vi "test_extended_audio.vi"() -> ()   [LabVIEW 2023]
panel:
  out "Waveform Chart":sgl[](graph)
  in  "stop":bool
  in  "host":string="192.168.1.7"
  in  "path in":path=path "C:/Users/jcds/Documents/GitHub/hl2ss/extensions/client_labview/hl2ss_labview/hl2ss_ulm.dll"
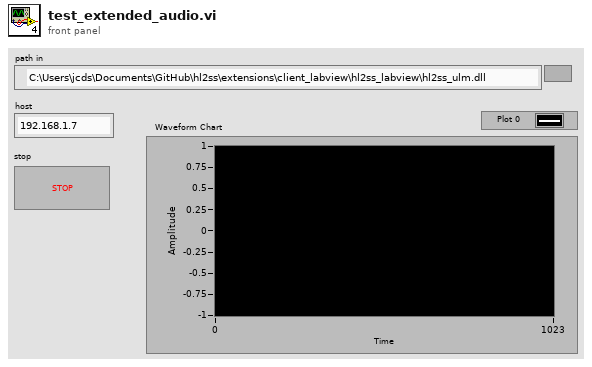
[diagram p1: front panel]
types:
  T1 = cluster{"chunk":u64, "mixer_mode":u32, "loopback_gain":sgl, "microphone_gain":sgl, "profile":u8, "level":u8, "_reserved_0":u8, "_reserved_1":u8}
  T2 = cluster{"frame_stamp":i64, "timestamp":u64, "payload_size":u32, "status":i32, "payload":u64, "pose":u64}
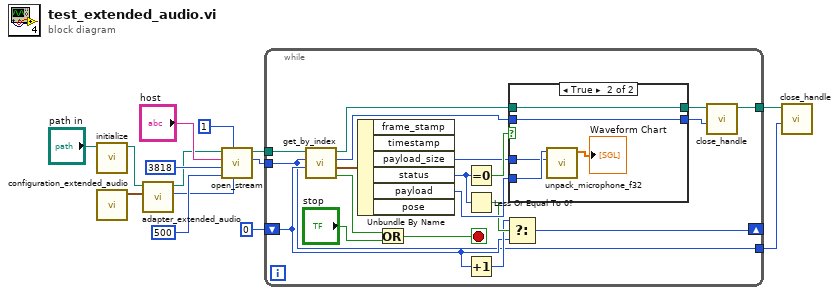
[diagram p0: block diagram]
diagram:
  n1 = call "initialize.vi"("path in"="path in") -> ("path out"=w4:path)  [unwired: 9 in, 1 out]
  n2 = call "configuration_extended_audio.vi"() -> ("configuration_extended_audio"=w5:T1)  [unwired: 11 in]
  n3 = call "adapter_extended_audio.vi"("configuration_extended_audio"=w5, "path in"=w4) -> ("configuration"=w2:u64, "path out"=w3:path)  [unwired: 8 in]
  n4 = call "open_stream.vi"("configuration"=w2, "decoded"=u8 1, "buffer_size"=u64 500, "port"=u16 3818, "host"="host", "path in"=w3) -> ("handle"=w13:u64, "path out"=w12:path)  [unwired: 3 in, 1 out]
  n5 = while {
    shift-right: [w26] -> _
    shift-left: i64 0 ("status") -> [w27]
    tunnel: w13 -> [w19]
    tunnel: w12 -> [w25]
    tunnel: [w20] -> w7
    tunnel: [w19] -> w6
    stop <- w18 stop-if-true
    n6 = call "get_by_index.vi"("frame_stamp"=w27, "stream_handle"=w19, "path in"=w25) -> ("error"=w17:bool, "packet"=w33:T2, "packet_handle"=w23:u64, "path out"=w24:path)  [unwired: 5 in]
    n7 = Unbundle By Name(w33) -> ("payload_size"=w15:u32, "status"=w30:i32, "payload"=w31:u64)  [unwired: 3 out]
    n8 = Or(x=w17, y="stop") -> (x .or. y?=w18:bool)
    n9 = Equal To 0?(x=w30) -> (x = 0?=w32:bool)
    n10 = Less Or Equal To 0?(x=w30) -> (x <= 0?=w29:bool)
    n11 = Increment(x=w27) -> (x+1=w28:i64)
    n12 = Select(t=w28, s=w29, f=w27) -> (s? t:f=w26:i64)
    n13 = case shown="True" w32 {
      tunnel: w31 -> [_ w38]
      tunnel: w24 -> [w35 w40]
      tunnel: w23 -> [w34 w39]
      tunnel: [w35 w40] -> w22
      tunnel: [w34 w39] -> w21
      tunnel: w15 -> [_ w37]
      frame False {
      }
      frame True {
        n14 = call "unpack_microphone_f32.vi"("payload_size"=w37, "payload"=w38) -> ("samples"=→"Waveform Chart":sgl[])  [unwired: 8 in, 1 out]
      }
    }
    n15 = call "close_handle.vi"("handle"=w21, "path in"=w22) -> ("path out"=w20:path)  [unwired: 9 in]
  }
  n16 = call "close_handle.vi"("handle"=w6, "path in"=w7) -> ()  [unwired: 9 in, 1 out]
